vi "Distance To Scanning Tank.vi"(3 "Move Z Distance (mm)":dbl, 4 "Move Y Distance (mm)":dbl, 5 "Move X Distance (mm)":dbl) -> (0 "Z Steps":string, 1 "Y Steps":string, 2 "X Steps":string)   [LabVIEW 2020]
doc: "Groups the individual X,Y,Z distance to step conversion into one sub-vi for the purpose of moving to the starting scan point (i.e. distance to the scanning tank).\n\nArgs:\n\nMove X Distance (mm): Distance the user wants to move in the x direciton in the form of an integer\nMove Y Distance (mm): Distance the user wants to move in the y direciton in the form of an integer\nMove Z Distance (mm): Distance the user wants to move in the z direciton in the form of an integer\n\nReturns:\n\nX Steps: Number of steps required to achieve the input X distance in the form of a string\nY Steps: Number of steps required to achieve the input Y distance in the form of a string\nZ Steps: Number of steps required to achieve the input Z distance in the form of a string"
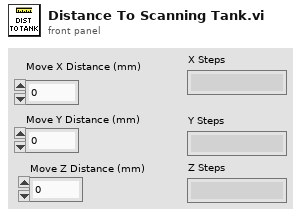
[diagram p1: front panel]
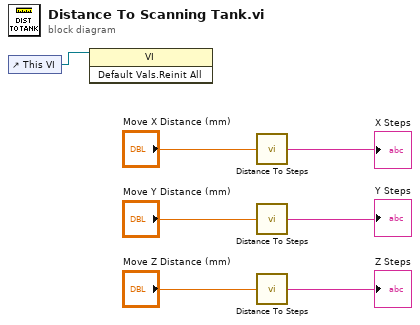
[diagram p0: block diagram]
diagram:
  n1 = control-ref of="This VI"() -> (w1:refnum<vi>)
  n2 = invoke class="VI" method="Default Vals.Reinit All"(reference=w1) -> ()  [unwired: 2 in, 3 out]
  n3 = call "Distance To Steps.vi"("Desired Distance (mm)"="Move X Distance (mm)") -> ("Number of Steps"=→"X Steps":string)
  n4 = call "Distance To Steps.vi"("Desired Distance (mm)"="Move Y Distance (mm)") -> ("Number of Steps"=→"Y Steps":string)
  n5 = call "Distance To Steps.vi"("Desired Distance (mm)"="Move Z Distance (mm)") -> ("Number of Steps"=→"Z Steps":string)
